vi "Build Full GIC B.vi"(6 "Parameters":dbl[](array[numeric]), 7 "Sim Course":i8[][](array[numeric]), 8 "Obst Lats and Longs":cluster{"Obst Lats":dbl[], "Obst Longs":dbl[]} {"Obst Longs" format="%#_8g"; "Obst Lats" format="%#_8g"}, 9 "WP Lats and Longs":cluster{"WP Lats":dbl[], "WP Longs":dbl[]}, 10 "Num of WPs":i16, 11 "?":T3={"     Use ?\nOff       On"=[FALSE, TRUE, FALSE, TRUE], "Mode:"=FALSE, "Extra Port"="", "Hokuyo Port"="COM7", "Tx Prop  Port"="COM6", "Compass Port"="", "GPS Port"=""}) -> (3 "Full GIC":T1={"     Use ?\nOff       On"=[FALSE, TRUE, FALSE, TRUE], "Mode:"=FALSE, "Extra Port"="", "Hokuyo Port"="COM7", "Tx Prop  Port"="COM6", "Compass Port"="", "GPS Port"="", "Num of WPs"=0, "WP Lats and Longs"={"WP Lats"=[], "WP Longs"=[]}, "Obst Lats and Longs"={"Obst Lats"=[], "Obst Longs"=[]}, "Parameters"=[], "GPS Data"=[], "Compass"=0.0, "LMS Vector"=[], "Vision Vector"=[], "Direction Cmd"=0.0, "Speed Cmd"=0.0, "WP Vector"=[], "WP Number"=0, "Extra"=0, "SW Map"=[], "Path Cluster"={"Path x node"=[], "Path y node"=[]}, "Sim Course"=[]} {"Obst Lats and Longs"."Obst Longs" format="%#_8g"; "Obst Lats and Longs"."Obst Lats" format="%#_8g"})   [LabVIEW 2014]
panel:
  in  "Path Cluster":T2
  in  "Extra":i16
  in  "WP Number":i32
  in  "WP Vector":dbl[](array[numeric])
  in  "Speed Cmd":dbl
  in  "Direction Cmd":dbl
  in  "GPS Data":dbl[](array[numeric])
  in  "Compass":dbl
  # "Build Full GIC B"
  # "SetUp GIC Elements"
  # "Items from Top VI"
  # "Add these to GIC"
  # "Output Full GIC"
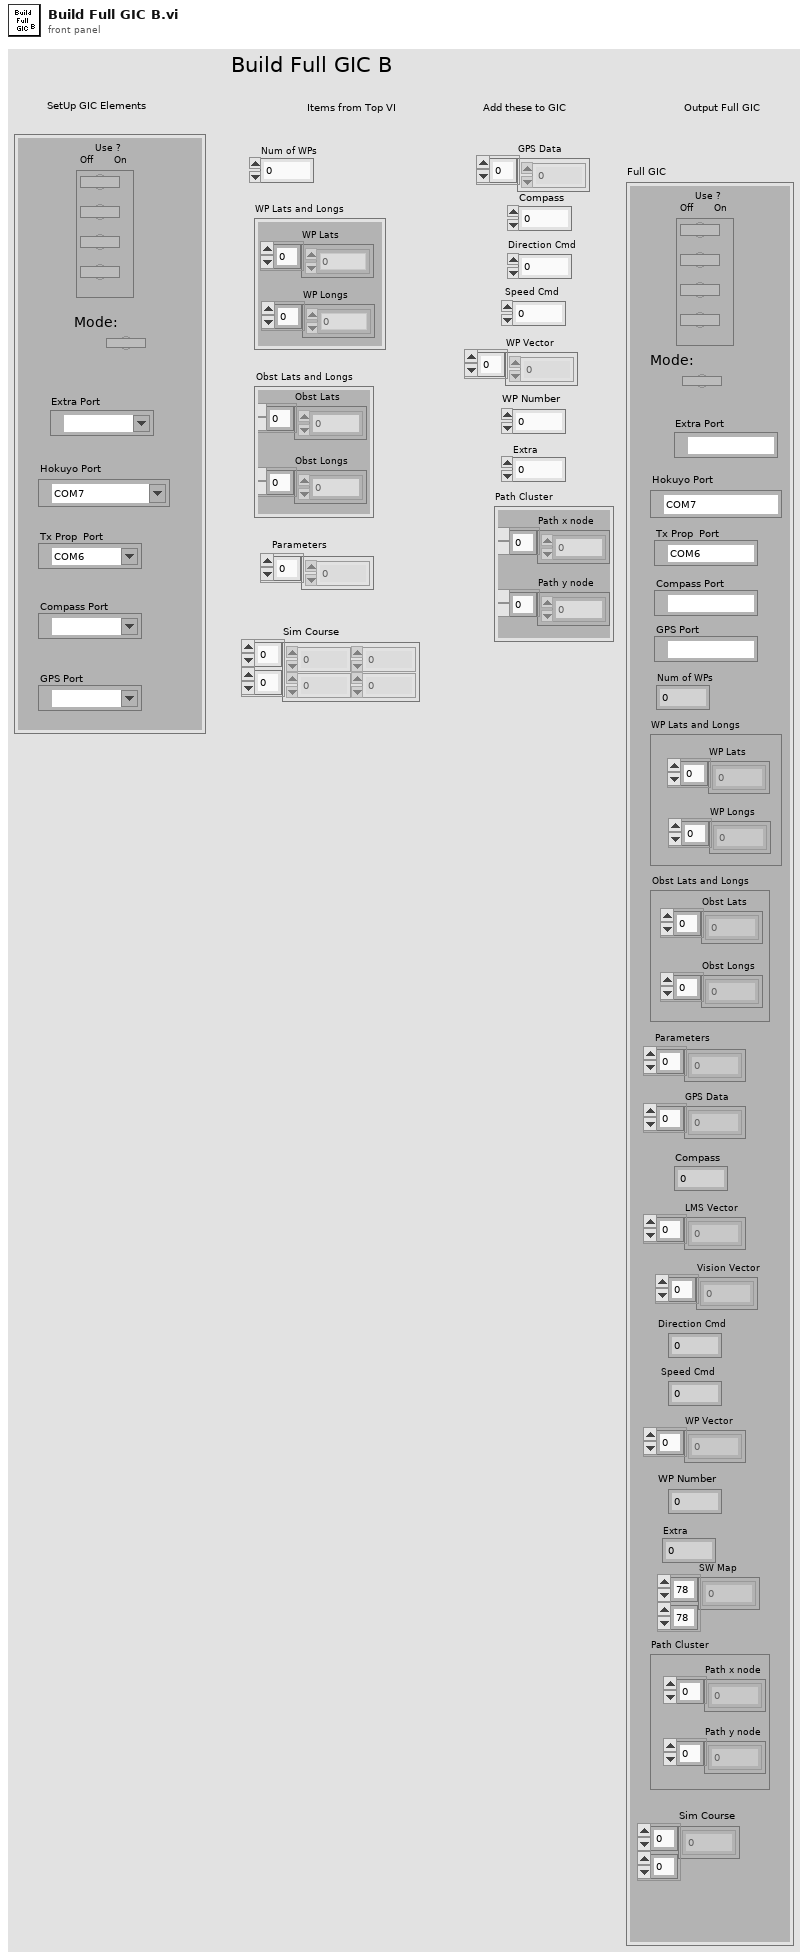
[diagram p1: front panel]
types:
  T1 = cluster{"     Use ?\nOff       On":bool[], "Mode:":bool, "Extra Port":refnum<visa-resource-name>, "Hokuyo Port":refnum<visa-resource-name>, "Tx Prop  Port":refnum<visa-resource-name>, "Compass Port":refnum<visa-resource-name>, "GPS Port":refnum<visa-resource-name>, "Num of WPs":i16, "WP Lats and Longs":cluster{"WP Lats":dbl[], "WP Longs":dbl[]}, "Obst Lats and Longs":cluster{"Obst Lats":dbl[], "Obst Longs":dbl[]}, "Parameters":dbl[], "GPS Data":dbl[], "Compass":dbl, "LMS Vector":dbl[], "Vision Vector":dbl[], "Direction Cmd":dbl, "Speed Cmd":dbl, "WP Vector":dbl[], "WP Number":i32, "Extra":i16, "SW Map":i32[][], "Path Cluster":cluster{"Path x node":dbl[], "Path y node":dbl[]}, "Sim Course":i8[][]}
  T2 = cluster{"Path x node":dbl[], "Path y node":dbl[]}
  T3 = cluster{"     Use ?\nOff       On":bool[], "Mode:":bool, "Extra Port":refnum<visa-resource-name>, "Hokuyo Port":refnum<visa-resource-name>, "Tx Prop  Port":refnum<visa-resource-name>, "Compass Port":refnum<visa-resource-name>, "GPS Port":refnum<visa-resource-name>}
  T4 = cluster{"     Use ?\nOff       On":bool[], "Mode:":bool, "Extra Port":refnum<visa-resource-name>, "Hokuyo Port":refnum<visa-resource-name>, "Tx Prop  Port":refnum<visa-resource-name>, "Compass Port":refnum<visa-resource-name>, "GPS Port":refnum<visa-resource-name>, "Num of WPs":i16, "WP Lats and Longs":cluster{"WP Lats":dbl[], "WP Longs":dbl[]}, "Obst Lats and Longs":cluster{"Obst Lats":dbl[], "Obst Longs":dbl[]}, "Parameters":dbl[], "GPS Data":dbl[], "Compass":dbl, dbl[], dbl[], "Direction Cmd":dbl, "Speed Cmd":dbl, "WP Vector":dbl[], "WP Number":i32, "Extra":i16, dbl[][], "Path Cluster":cluster{"Path x node":dbl[], "Path y node":dbl[]}, "Sim Course":i8[][]}
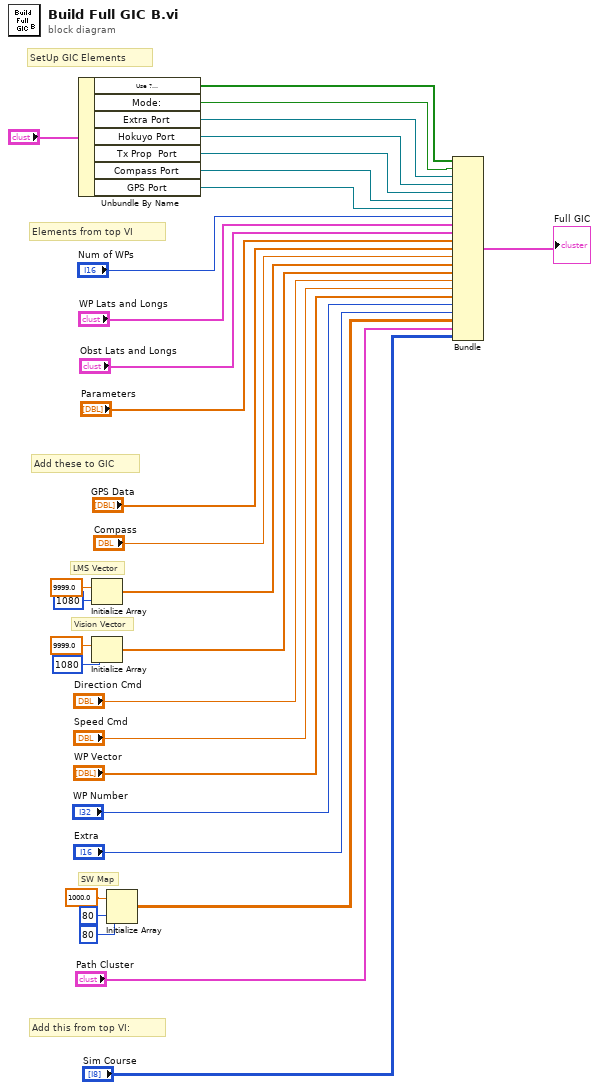
[diagram p0: block diagram]
diagram:
  # "Add this from top VI:"
  # "SW Map"
  # "Vision Vector"
  # "LMS Vector"
  # "Add these to GIC"
  # "Elements from top VI"
  # "SetUp GIC Elements"
  n1 = Unbundle By Name("?") -> ("Use ?\nOff       On"=w3:bool[], "Mode:"=w4:bool, "Extra Port"=w5:refnum<visa-resource-name>, "Hokuyo Port"=w6:refnum<visa-resource-name>, "Tx Prop  Port"=w24:refnum<visa-resource-name>, "Compass Port"=w23:refnum<visa-resource-name>, "GPS Port"=w22:refnum<visa-resource-name>)
  n2 = Initialize Array(9999.0 ("element"), 1080 ("dimension size")) -> (w15:dbl[])
  n3 = Initialize Array(9999.0 ("element"), 1080 ("dimension size")) -> (w14:dbl[])
  n4 = Initialize Array(1000.0 ("element"), 80 ("dimension size"), 80 ("dimension size")) -> (w8:dbl[][])
  n5 = Bundle("Use ?\nOff       On"=w3, "Mode:"=w4, "Extra Port"=w5, "Hokuyo Port"=w6, "Tx Prop  Port"=w24, "Compass Port"=w23, "GPS Port"=w22, "Num of WPs"="Num of WPs", "WP Lats and Longs"="WP Lats and Longs", "Obst Lats and Longs"="Obst Lats and Longs", "Parameters"="Parameters", "GPS Data"="GPS Data", "Compass"="Compass", w15, w14, "Direction Cmd"="Direction Cmd", "Speed Cmd"="Speed Cmd", "WP Vector"="WP Vector", "WP Number"="WP Number", "Extra"="Extra", w8, "Path Cluster"="Path Cluster", "Sim Course"="Sim Course") -> (→"Full GIC":T4)  [unwired: 1 in]
